vi "Get Data.vi"(8 "error in":errorcluster, 11 "PAS in":refnum<class "PAS.lvclass">) -> (0 "error out":errorcluster, 3 "PAS out":refnum<class "PAS.lvclass">)   [LabVIEW 2014, in "PAS.lvclass"]
doc: "Here you will do all of your acquisition. The acquisition is going to be implementation dependent, but at the bare minimum the class which inherits the PAS will have to retrieve the speaker signal(s). The data that is acquired in this cycle will be piped to the <b>Analyze Data</b> VI in the next cycle."
uses:
  PAS.lvclass
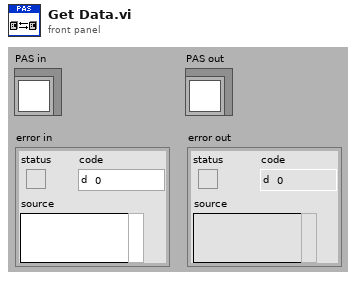
[diagram p1: front panel]
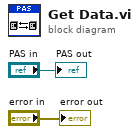
[diagram p0: block diagram]
diagram:
  "error out" <- "error in"
  "PAS out" <- "PAS in"
